vi "AutoProgram.vi"(0 "G-Code Array":string[](array[string]), 2 "INcluster":T1, 4 "error in (no error)":errorcluster) -> (5 "Next Command":string, 6 "Stop State":bool, 7 "error out":errorcluster)   [LabVIEW 2017]
uses:
  controls/QueueControl.ctl
  controls/CommandQueue.ctl
panel:
  out "# elements in queue":i32
  in  "STATE BOARD":enum16{"Running", "Waiting", "Pos", "IDLE"}(ring)
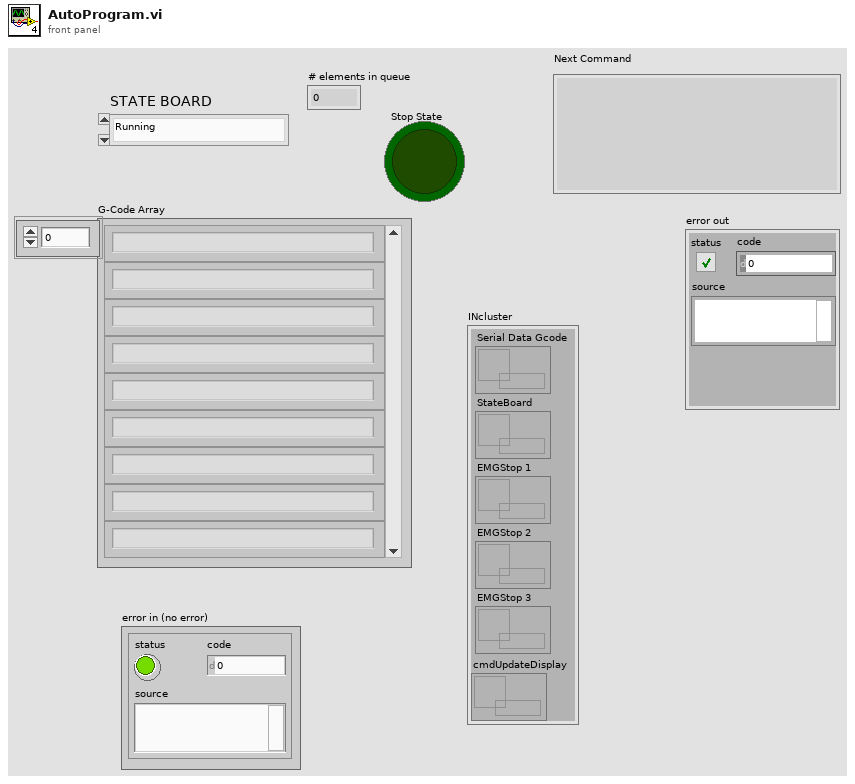
[diagram p1: front panel]
types:
  T1 = typedef "QueueControl.ctl" = cluster{"Serial Data Gcode":refnum<queue>, "StateBoard":refnum<queue>, "EMGStop 1":refnum<queue>, "EMGStop 2":refnum<queue>, "EMGStop 3":refnum<queue>, "cmdUpdateDisplay":refnum<queue>}
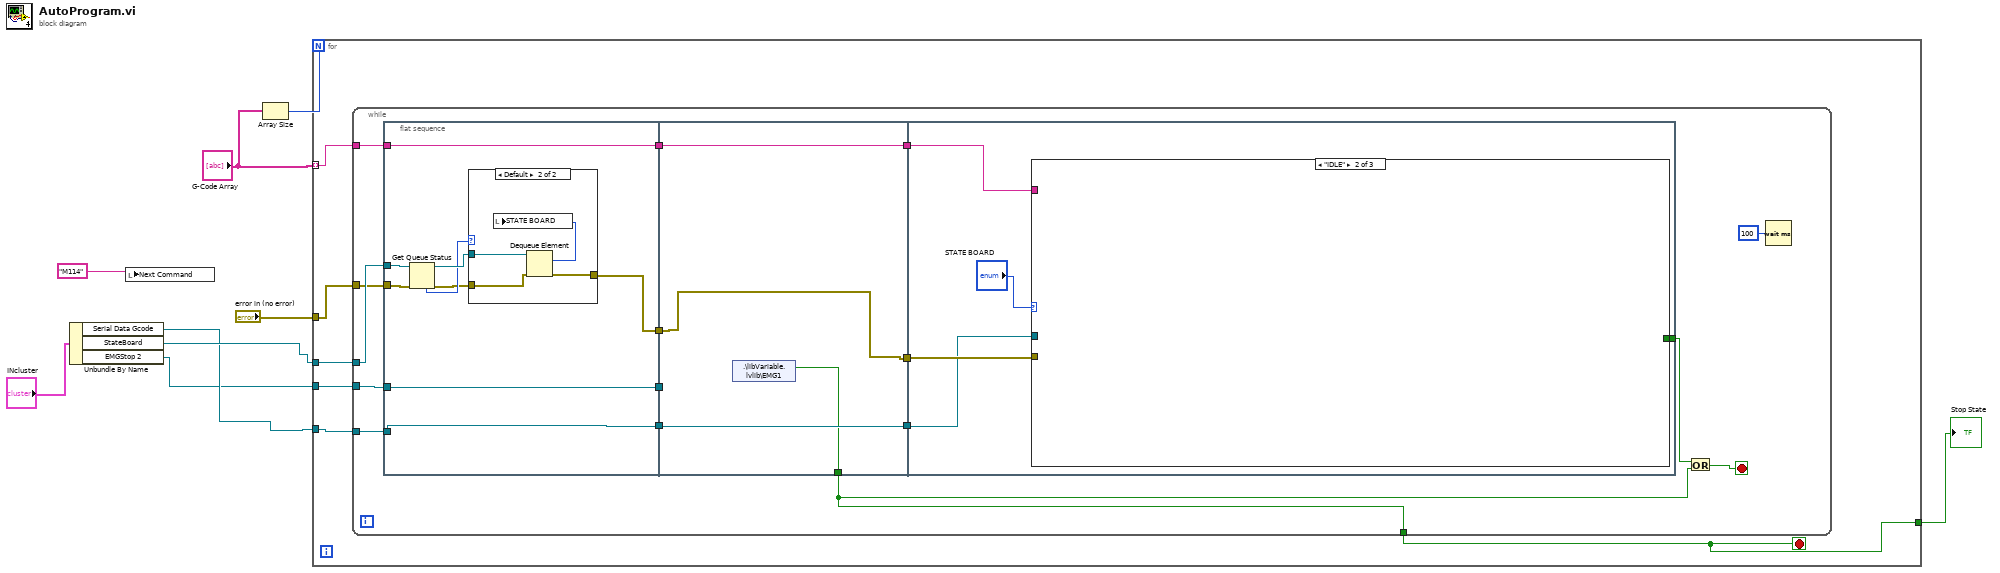
[diagram p0: block diagram]
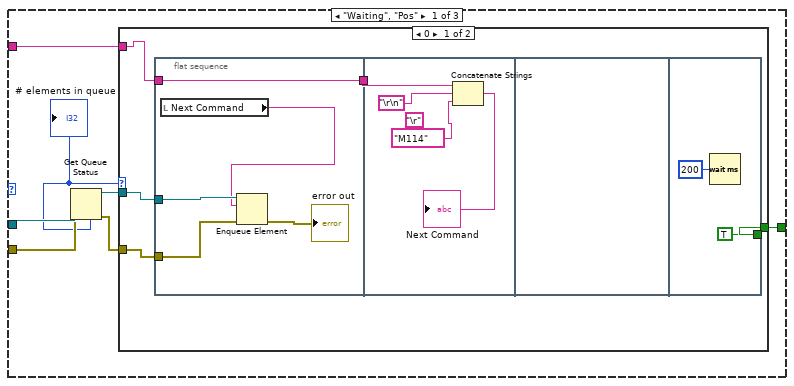
[diagram p3: hidden frame]
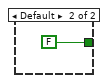
[diagram p4: hidden frame]
diagram:
  n1 = Unbundle By Name("INcluster") -> ("Serial Data Gcode"=w5:refnum<queue>, "StateBoard"=w6:refnum<queue>, "EMGStop 2"=w1:refnum<queue>)
  n2 = local write "Next Command"("M114" ("Next Command")) -> ()
  n3 = Array Size(array="G-Code Array") -> (size(s)=w9:i32)
  n4 = for {
    N: w9 -> [_]
    tunnel: "G-Code Array" -> [w11] mode=indexing
    tunnel: "error in (no error)" -> [w15]
    tunnel: w5 -> [w12]
    tunnel: w6 -> [w14]
    tunnel: w1 -> [w13]
    tunnel: [w10] -> w4
    stop <- w10 stop-if-true
    n5 = while {
      tunnel: w15 -> [w28]
      tunnel: [w26] -> w10
      tunnel: w14 -> [w29]
      tunnel: w13 -> [w23]
      tunnel: w12 -> [w20]
      tunnel: w11 -> [w18]
      stop <- w30 stop-if-true
      n6 = flat-sequence {
        tunnel: w29 -> [w40]
        tunnel: w28 -> [w37]
        tunnel: [w35] -> w25
        tunnel: [w34] -> w24
        tunnel: w23 -> [w34]
        tunnel: [w33] -> w21
        tunnel: w20 -> [w33]
        tunnel: w18 -> [w32]
        tunnel: [w32] -> w17
        tunnel: [w47] -> w27
        tunnel: [w46] -> w26
        tunnel: w25 -> [w47]
        tunnel: w24 -> [_]
        tunnel: [w49] -> w22
        tunnel: w21 -> [w49]
        tunnel: w17 -> [w48]
        tunnel: [w48] -> w16
        tunnel: w27 -> [w54]
        tunnel: [w53] -> w19
        tunnel: w22 -> [w50]
        tunnel: w16 -> [w51]
        frame #0 {
          n7 = Get Queue Status(queue=w40, error in (no error)=w37) -> (queue out=w39:refnum<queue>, error out=w36:errorcluster, # elements in queue=w38:i32)  [unwired: 1 in, 5 out]
          n8 = case shown="Default" w38 {
            tunnel: w39 -> [_ w44]
            tunnel: w36 -> [w41 w43]
            tunnel: [w41 w42] -> w35
            frame 0 {
            }
            frame Default {
              n9 = Dequeue Element(queue=w44, error in (no error)=w43) -> (element=w45:enum16{"Running", "Waiting", "Pos", "IDLE"}, error out=w42:errorcluster)  [unwired: 1 in, 2 out]
              n10 = local write "STATE BOARD"(w45) -> ()
            }
          }
        }
        frame #1 {
          n11 = shared-variable ".\\libVariable.lvlib\\EMG1"() -> (w46:bool)  [unwired: 1 in, 1 out]
        }
        frame #2 {
          n12 = case shown="\"IDLE\"" "STATE BOARD" {
            tunnel: w50 -> [w59 _ _]
            tunnel: w54 -> [w57 _ _]
            tunnel: w51 -> [w60 _ _]
            tunnel: [w61 _ _] -> w53
            frame "Waiting", "Pos" {
              n13 = Get Queue Status(queue=w59, error in (no error)=w57) -> (queue out=w58:refnum<queue>, error out=w56:errorcluster, # elements in queue=w55:i32)  [unwired: 1 in, 5 out]
              "# elements in queue" <- w55
              n14 = case shown="0" w55 {
                tunnel: [w65 FALSE] -> w61
                tunnel: w60 -> [w62 _]
                tunnel: w58 -> [w64 _]
                tunnel: w56 -> [w63 _]
                frame 0 {
                  n15 = flat-sequence {
                    tunnel: w63 -> [w71]
                    tunnel: w62 -> [w69]
                    tunnel: [w69] -> w66
                    tunnel: w64 -> [w68]
                    tunnel: w66 -> [w74]
                    tunnel: [TRUE] -> w65
                    frame #0 {
                      n16 = local read "Next Command"() -> (w67:string)
                      n17 = Enqueue Element(queue=w68, element=w67, error in (no error)=w71) -> (error out=→"error out":errorcluster)  [unwired: 1 in, 2 out]
                    }
                    frame #1 {
                      (unwired) "\r"
                      n18 = Concatenate Strings(w74, "\r\n", "M114" ("string")) -> (→"Next Command":string)
                    }
                    frame #2 {
                    }
                    frame #3 {
                      n19 = Wait (ms)(milliseconds to wait=u32 200) -> ()  [unwired: 1 out]
                    }
                  }
                }
                frame Default {
                }
              }
            }
            frame "IDLE" {
            }
            frame "Running" {
            }
          }
        }
      }
      n20 = Or(x=w19, y=w26) -> (x .or. y?=w30:bool)
      n21 = Wait (ms)(milliseconds to wait=u32 100) -> ()  [unwired: 1 out]
    }
  }
  "Stop State" <- w4
